vi "Configure Measurement (Adjacent Channel Power Ratio Filter).vi"(0 "VISA resource name":refnum<visa-resource-name>, 5 "Enable RRC Filter (F: Disable)":bool, 9 "RRC Filter Alpha Value (0.01)":dbl=0.01, 11 "error in (no error)":errorcluster) -> (4 "VISA resource name out":refnum<visa-resource-name>, 15 "error out":errorcluster)   [LabVIEW 2022 SP3, in "Agilent N934X Series.lvlib"]
doc: "Configures the filter settings of ACPR measurement type.\n\nNote:\nThis VI is only applicable for N9321C, N9322C, N9323C, N9324C models."
uses:
  <instrlib>/Agilent N934X Series/Agilent N934X Series.lvlib
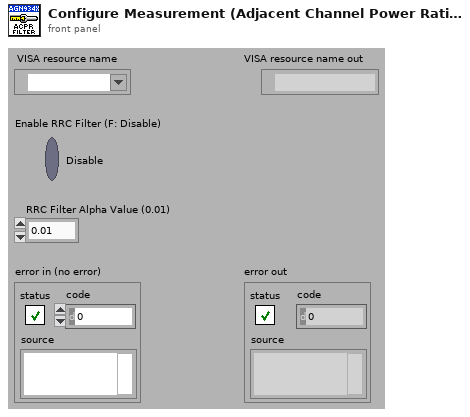
[diagram p1: front panel]
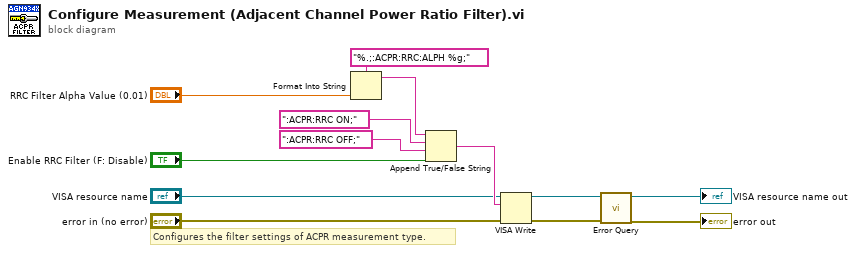
[diagram p0: block diagram]
diagram:
  # "Configures the filter settings of ACPR measurement type."
  n1 = Format Into String(format string="%.;:ACPR:RRC:ALPH %g;", "RRC Filter Alpha Value (0.01)") -> (resulting string=w11:string)  [unwired: 2 in, 1 out]
  n2 = Append True/False String(1:"Enable RRC Filter (F: Disable)", 2:":ACPR:RRC OFF;", 3:":ACPR:RRC ON;", 4:w11) -> (0:w7:string)
  n3 = VISA Write(VISA resource name="VISA resource name", write buffer=w7, error in (no error)="error in (no error)") -> (VISA resource name out=w4:refnum<visa-resource-name>, error out=w3:errorcluster)  [unwired: 1 out]
  n4 = call <instrlib>:"Error Query.vi"("error in (no error)"=w3, "VISA resource name"=w4) -> ("error out"=→"error out":errorcluster, "VISA resource name out"=→"VISA resource name out":refnum<visa-resource-name>)  [unwired: 6 in, 2 out]
